vi "BoxString.vi"(10 "String":string) -> (2 "String out":refnum<class "String.lvclass">)   [LabVIEW 2017, in "LapDog.Collections.v0.Lists.Interfaces.lvlib" / "String.lvclass"]
uses:
  String.lvclass
  String.lvclass/String.ctl
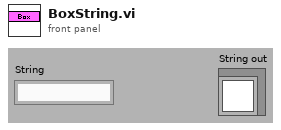
[diagram p1: front panel]
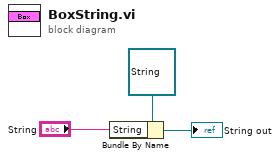
[diagram p0: block diagram]
diagram:
  n1 = Bundle By Name(cluster=refnum<class "String.lvclass"> refnum ("LapDog.Collections.v0.Lists.Interfaces.lvlib:String.lvclass"), "String"="String") -> (→"String out":refnum<class "String.lvclass">)
